vi "NI-DCPower Sink DC Current + Ammeter.vi"() -> ()   [LabVIEW 2020]
doc: "Demonstrates how to use the DC Voltage Output Function to force an output voltage. This example initializes a session, configures the Output Function, Sense, Autorange, Voltage Level and Current Limit, initiates generation, waits for a specified delay, and measures the voltage and current output. This example uses Single Point source mode."
uses:
  <instrlib>/niDCPower/nidcpower.llb/niDCPower Sense.ctl
  <instrlib>/niDCPower/nidcpower.llb/niDCPower Source Mode.ctl
  <instrlib>/niDCPower/nidcpower.llb/niDCPower Output Function.ctl
  <instrlib>/niDCPower/nidcpower.llb/niDCPower Wait For Event - Event.ctl
panel:
  in  "Aperture Time (Sec)":dbl=0.01 format="%.3p"
  in  "Voltage Sense":T1=1009 caption="sense" items=["Local"=1008, "Remote"=1009]
  in  "Stop":bool
  in  "Source Delay (Sec)":dbl=0.01 format="%.3p"
  out "Voltage Measurement":dbl
  out "Current Measurement":dbl
  out "Compliance/Limit Reached":bool
  in  "Voltage Limit":dbl=6.0 caption="Current Limit" format="%.3p"
  in  "Current Level":dbl=1.0 caption="Voltage Level" format="%.5p"
  in  "Channel Name":string="0"
  in  "Resource Name":refnum<k15>="Dev1"
  # "Overview: Demonstrates how to use the DC Current Output Function to sink an input current.  \nThis example initializes a session; configures the Output Function, Voltage Limit and Current Level; \ninitiates generation; waits for a specified delay; and measures the voltage and current output. \nRequirements: NI-DCPower\nInstructions:\n1. Select the appropriate device in the Resource Name control.\n2. Configure the parameters of the DC Current signal you'd like to output.\n3. Run the VI."
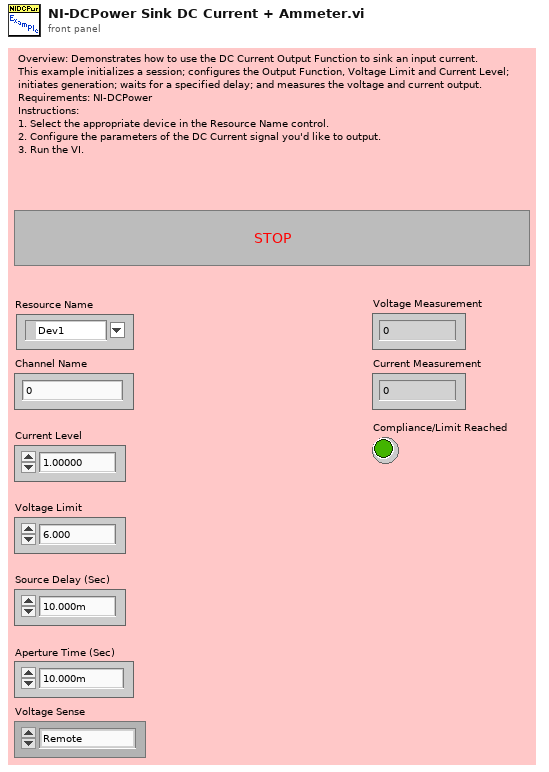
[diagram p1: front panel]
types:
  T1 = typedef "niDCPower Sense.ctl" = i32
  T2 = typedef "niDCPower Output Function.ctl" = i32
  T3 = typedef "niDCPower Source Mode.ctl" = i32
  T4 = typedef "niDCPower Wait For Event - Event.ctl" = i32
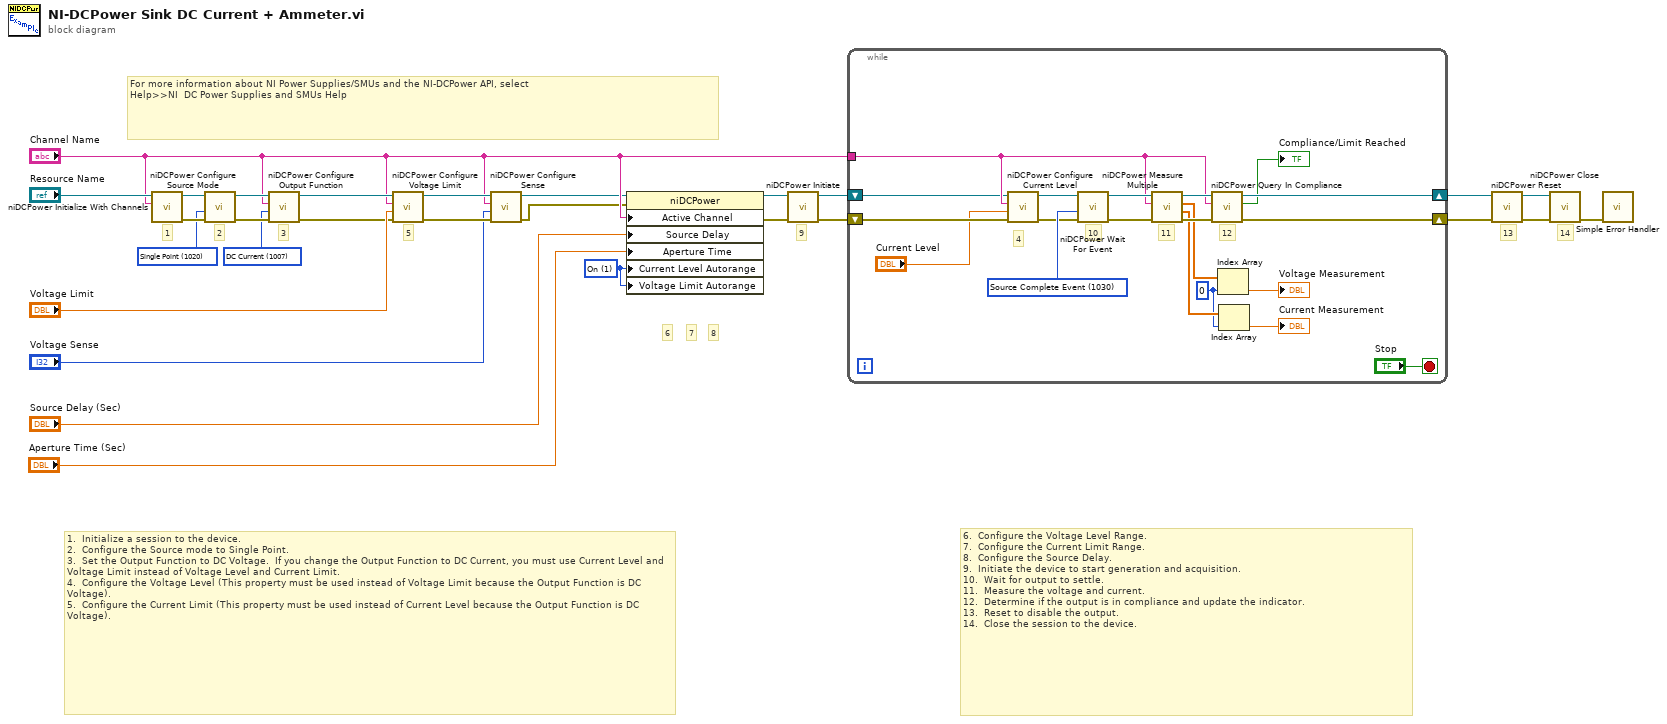
[diagram p0: block diagram]
diagram:
  w2 = 1 items=["Off", "On"] ("Source:DC Voltage:Voltage Level Autorange")
  w11 = T2 1007 items=["DC Voltage"=1006, "DC Current"=1007, "Pulse Voltage"=1049, "Pulse Current"=1050] ("output function")
  w17 = T3 1020 items=["Single Point"=1020, "Sequence"=1021] ("source mode")
  # "For more information about NI Power Supplies/SMUs and the NI-DCPower API, select\nHelp>>NI  DC Power Supplies and SMUs Help"
  # "14"
  # "9"
  # "7"
  # "6"
  # "2"
  # "1.  Initialize a session to the device.\n2.  Configure the Source mode to Single Point.\n3.  Set the Output Function to DC Voltage.  If you change the Output Function to DC Current, you must use Current Level and Voltage Limit instead of Voltage Level and Current Limit.\n4.  Configure the Voltage Level (This property must be used instead of Voltage Limit because the Output Function is DC Voltage).\n5.  Configure the Current Limit (This property must be used instead of Current Level because the Output Function is DC Voltage)."
  # "3"
  # "6.  Configure the Voltage Level Range.\n7.  Configure the Current Limit Range.\n8.  Configure the Source Delay.\n9.  Initiate the device to start generation and acquisition.\n10.  Wait for output to settle.\n11.  Measure the voltage and current.\n12.  Determine if the output is in compliance and update the indicator.\n13.  Reset to disable the output.\n14.  Close the session to the device."
  # "13"
  # "8"
  # "5"
  # "1"
  n1 = call <instrlib>:"niDCPower Initialize With Channels.vi"("channels"="Channel Name", "resource name"="Resource Name") -> ("error out"=w21:errorcluster, "instrument handle out"=w20:refnum<k15>)  [unwired: 3 in, 5 out]
  n2 = call <instrlib>:"niDCPower Configure Source Mode.vi"("error in (no error)"=w21, "source mode"=w17, "instrument handle"=w20) -> ("error out"=w19:errorcluster, "instrument handle out"=w18:refnum<k15>)  [unwired: 7 out]
  n3 = call <instrlib>:"niDCPower Configure Output Function.vi"("error in (no error)"=w19, "output function"=w11, "channel name"="Channel Name", "instrument handle"=w18) -> ("error out"=w9:errorcluster, "instrument handle out"=w10:refnum<k15>)  [unwired: 6 out]
  n4 = call <instrlib>:"niDCPower Configure Voltage Limit.vi"("error in (no error)"=w9, "voltage limit"="Voltage Limit", "channel name"="Channel Name", "instrument handle"=w10) -> ("error out"=w7:errorcluster, "instrument handle out"=w8:refnum<k15>)  [unwired: 6 in]
  n5 = call <instrlib>:"niDCPower Configure Sense.vi"("error in (no error)"=w7, "sense"="Voltage Sense", "channel name"="Channel Name", "instrument handle"=w8) -> ("error out"=w4:errorcluster, "instrument handle out"=w5:refnum<k15>)  [unwired: 6 in]
  n6 = property class="niDCPower"(reference=w5, error in=w4, "Active Channel"="Channel Name", "Source Delay"="Source Delay (Sec)", "Aperture Time"="Aperture Time (Sec)", "Current Level Autorange"=w2, "Voltage Limit Autorange"=w2) -> (reference out=w16:refnum<k15>, error out=w15:errorcluster)
  n7 = call <instrlib>:"niDCPower Initiate.vi"("error in (no error)"=w15, "instrument handle"=w16) -> ("error out"=w12:errorcluster, "instrument handle out"=w13:refnum<k15>)  [unwired: 2 in, 6 out]
  n8 = while {
    tunnel: "Channel Name" -> [w30]
    shift-right: [w48] -> w27
    shift-left: w13 -> [w29]
    shift-right: [w47] -> w24
    shift-left: w12 -> [w33]
    stop <- "Stop" stop-if-true
    w37 = T4 1030 items=["Source Complete Event"=1030, "Measure Complete Event"=1031, "Sequence Iteration Complete Event"=1032, "Sequence Engine Done Event"=1033] ("event")
    w42 = 0 ("index")
    # "4"
    # "11"
    # "10"
    # "12"
    n9 = call <instrlib>:"niDCPower Configure Current Level.vi"("error in (no error)"=w33, "current level"="Current Level", "channel name"=w30, "instrument handle"=w29) -> ("error out"=w34:errorcluster, "instrument handle out"=w35:refnum<k15>)  [unwired: 6 in]
    n10 = call <instrlib>:"niDCPower Wait For Event.vi"("error in (no error)"=w34, "event"=w37, "instrument handle"=w35) -> ("error out"=w38:errorcluster, "instrument handle out"=w39:refnum<k15>)  [unwired: 1 in, 6 out]
    n11 = call <instrlib>:"niDCPower Measure Multiple.vi"("error in (no error)"=w38, "channel name"=w30, "instrument handle"=w39) -> ("error out"=w45:errorcluster, "current measurements"=w43:dbl[], "voltage measurements"=w44:dbl[], "instrument handle out"=w46:refnum<k15>)  [unwired: 5 out]
    n12 = call <instrlib>:"niDCPower Query In Compliance.vi"("error in (no error)"=w45, "channel name"=w30, "instrument handle"=w46) -> ("error out"=w47:errorcluster, "in compliance?"=→"Compliance/Limit Reached":bool, "instrument handle out"=w48:refnum<k15>)  [unwired: 6 out]
    n13 = Index Array(array=w44, index=w42) -> (element=→"Voltage Measurement":dbl)
    n14 = Index Array(array=w43, index=w42) -> (element=→"Current Measurement":dbl)
  }
  n15 = call <instrlib>:"niDCPower Reset.vi"("error in (no error)"=w24, "instrument handle"=w27) -> ("error out"=w25:errorcluster, "instrument handle out"=w26:refnum<k15>)  [unwired: 2 in, 6 out]
  n16 = call <instrlib>:"niDCPower Close.vi"("error in (no error)"=w25, "instrument handle"=w26) -> ("error out"=w23:errorcluster)  [unwired: 9 out]
  n17 = call <vilib>:"Simple Error Handler.vi"("error in (no error)"=w23) -> ()  [unwired: 1 in, 8 out]
